vi "Launchtest.vi"(8 "error in (no error)":errorcluster, 11 "Operator name":string) -> (0 "error in (out)":errorcluster)   [LabVIEW 2024, in "LaunchTest.lvlib"]
doc: "This template is for the Queued Message Handler design pattern.\n\nThe Event Handling Loop generates messages based on user interface actions.\n\nThe Message Handling Loop processes messages generated by the Event Handling Loop, or by other messages. The messages are string values, so new messages can be added easily to the Message Cases case structure in the Message Handling Loop. Each message cluster can also provide an optional value for Message Data, which is a variant that can be converted to whatever message-specific data is required."
uses:
  LaunchTest.lvlib
  controls/Launch_UI Data.ctl
  PrivateControls/Launch_FGV_Queue_Control.ctl
  Test_2/TestMain2.vi
  <vilib>/Utility/error.llb/Error Cluster From Error Code.vi
  Launcher/MainLauncher.vi
  <vilib>/ErrorRing/Error Ring.xnode
  support/Message Queue/Launch_Message Queue.lvlib
  support/User Event - Stop/Launch_User Event - Stop.lvlib
  Launcher/Launcher_DTU.lvlib
  Test_2/Test_2.lvlib
  ADAM_DI/ADAM_DI.lvlib
panel:
  out "queue name 2":string
  out "queue name":string
  out "Display":string
  in  "Do Something Else <Replace Me>":bool
  in  "Do Something <Replace Me>":bool
  in  "Exit":bool
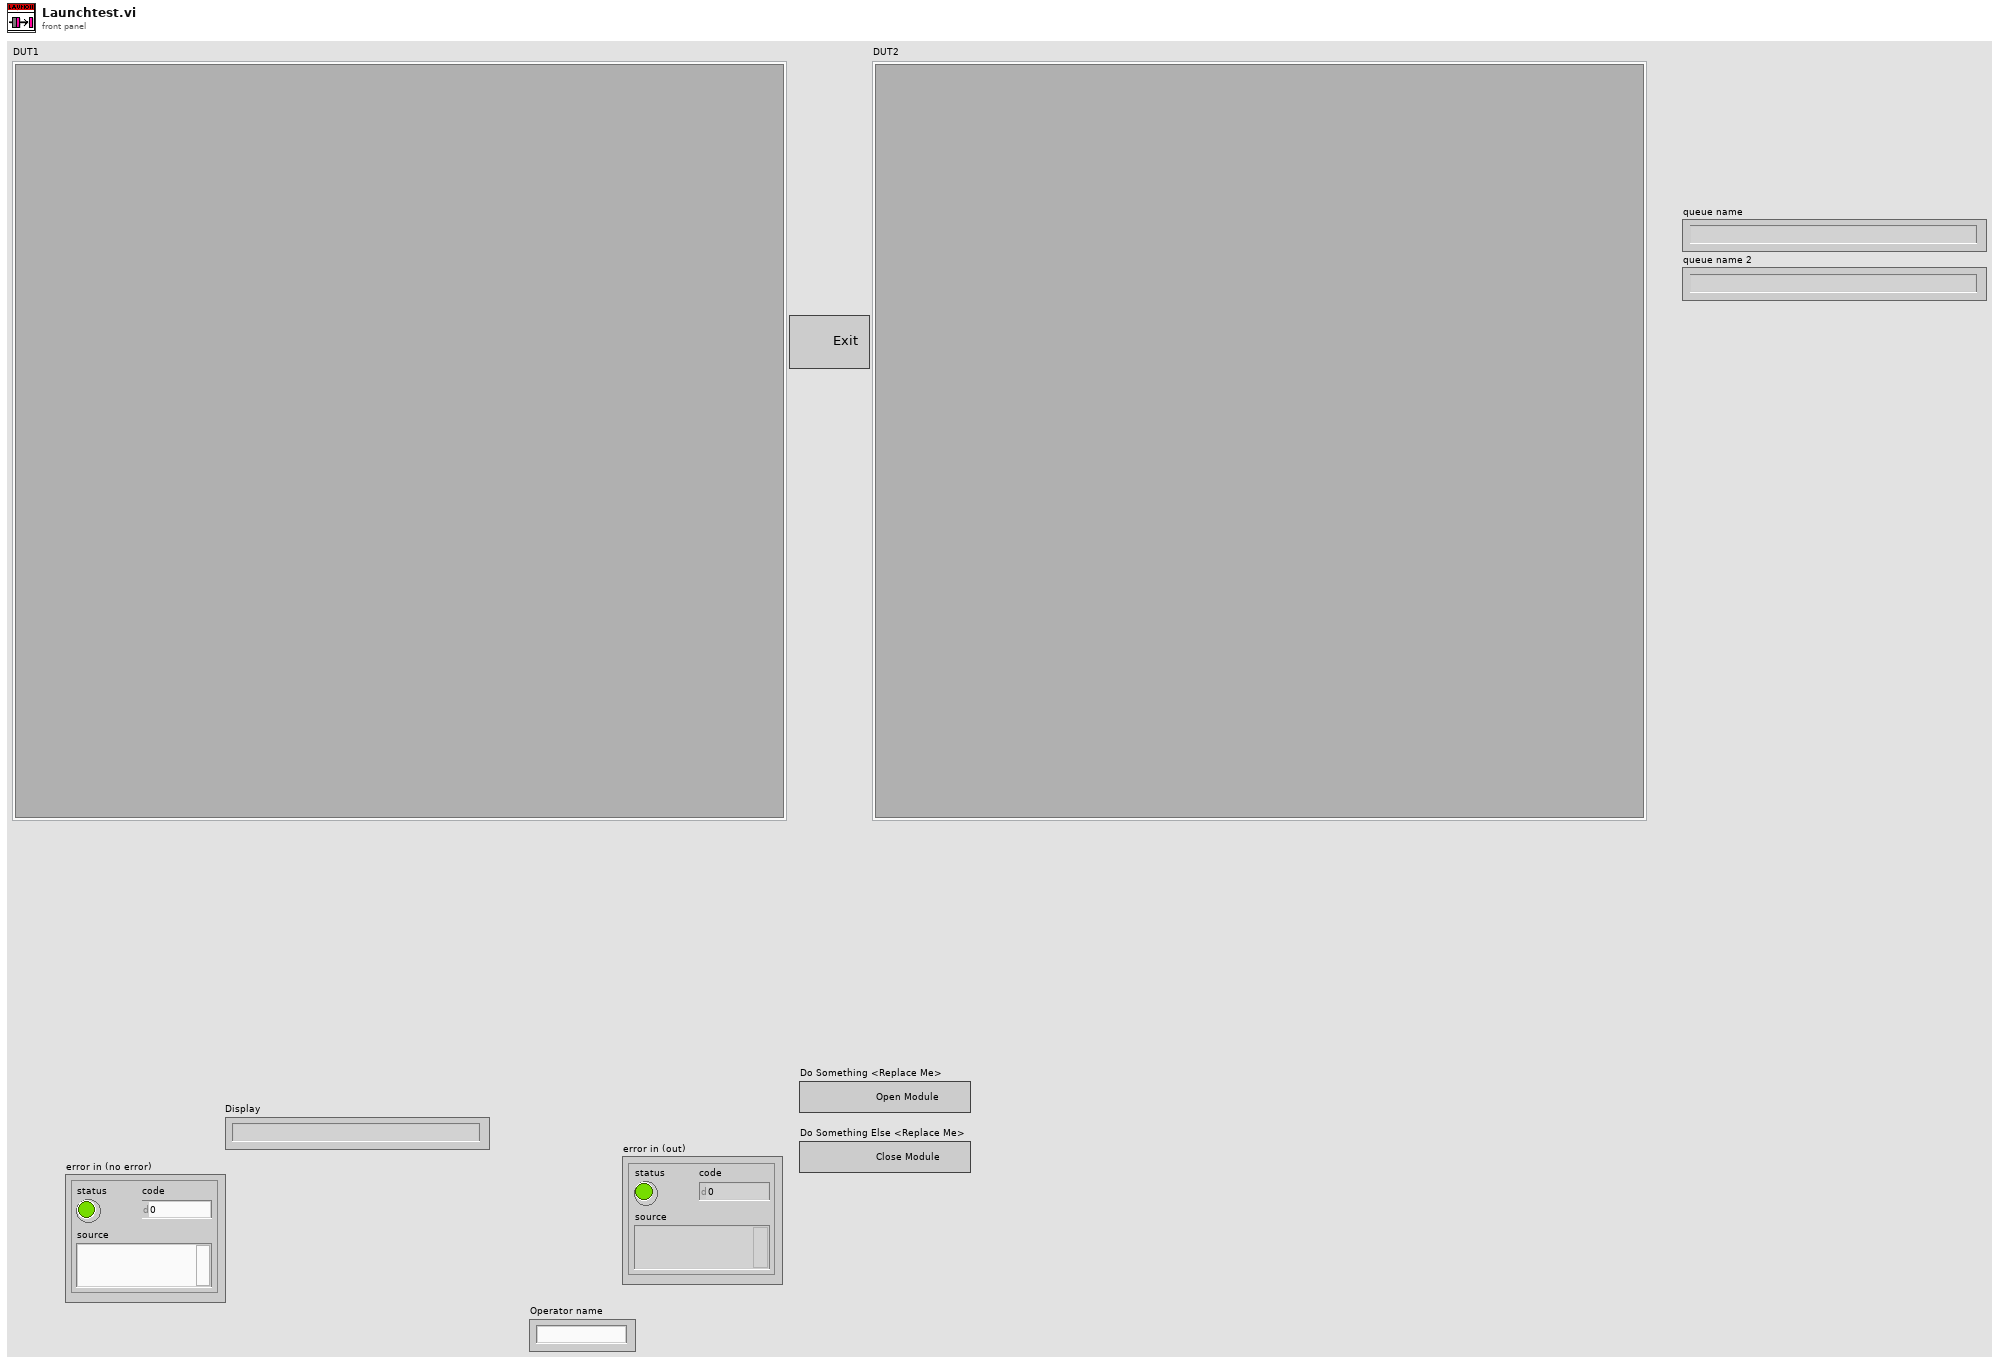
[diagram p1: front panel]
types:
  T1 = enum32{"Invalid", "Standard", "Closed", "Hidden", "Minimized", "Maximized"}
  T2 = typedef "LaunchTest.lvlib/Launch_FGV_Queue_Control.ctl" = enum16{"Release", "Get", "Set", "Flush"}
  T3 = typedef "LaunchTest.lvlib/Launch_UI Data.ctl" = cluster{"Launched?":bool, "Config":string, "Numeric <Replace Me>":dbl, "Operator":string, "Module path":path, "Config path":path, "Equip list":string[], "Test2_Q":refnum<queue>[], "CAMQ":refnum<queue>}
  T4 = typedef "LaunchTest.lvlib/Launch_Message Queue.lvlib/Launch_All Message Queues.ctl" = cluster{"UI":refnum<queue>, "QSM":refnum<queue>}
  T5 = enum16{"Read", "Write", "All_sections", "All_values", "Remove key&section"}
  T6 = cluster{"Message":string, "Message Data":variant}
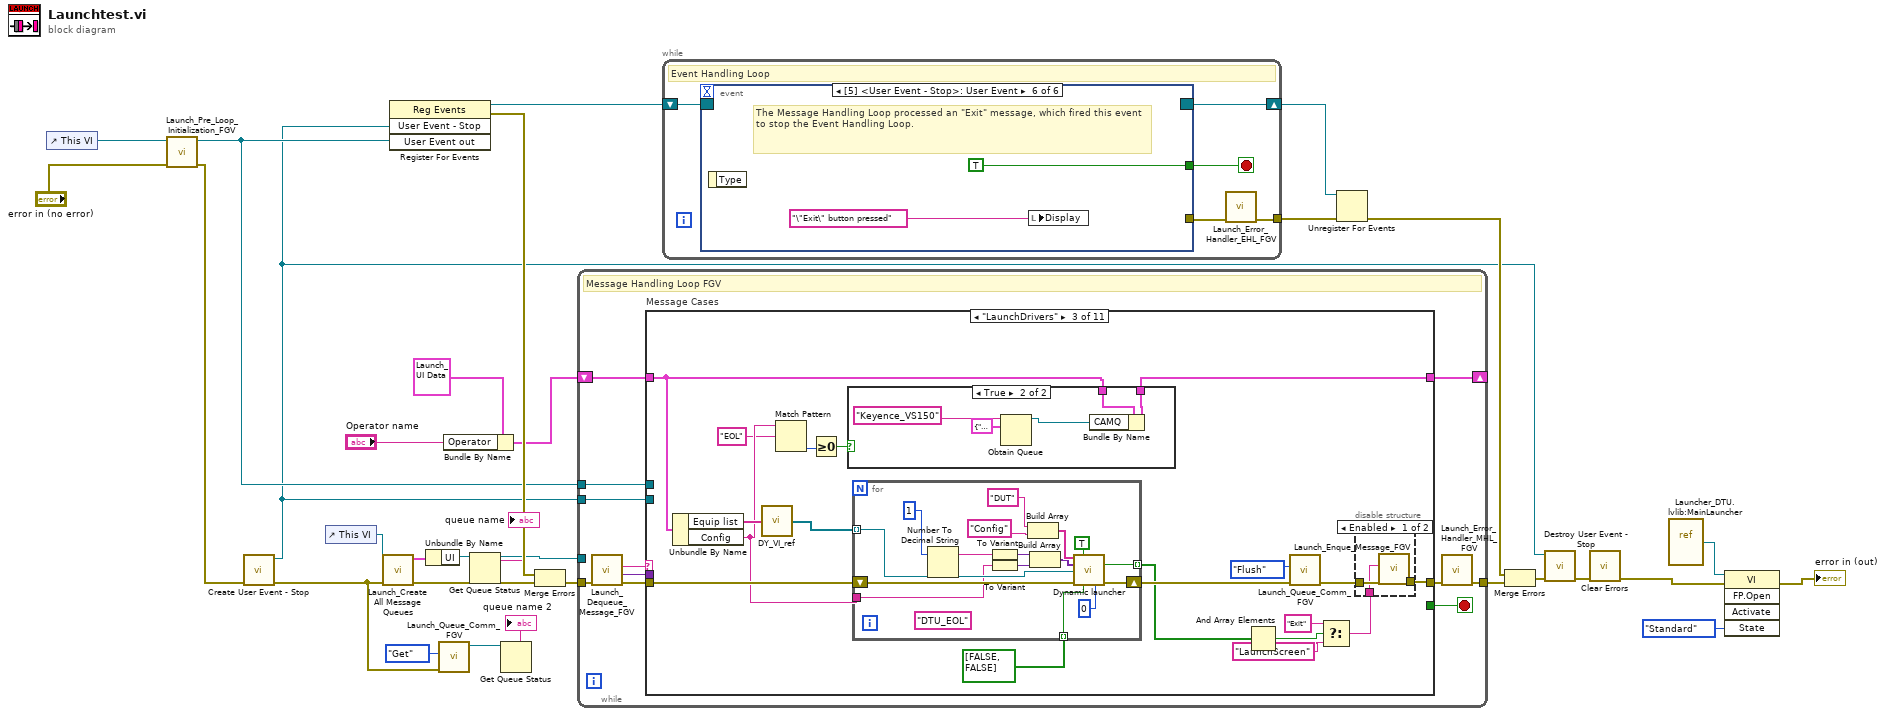
[diagram p0: block diagram]
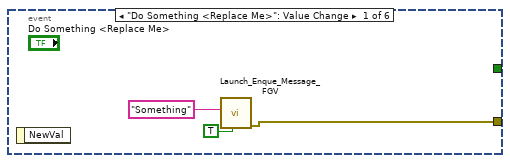
[diagram p2: hidden frame]
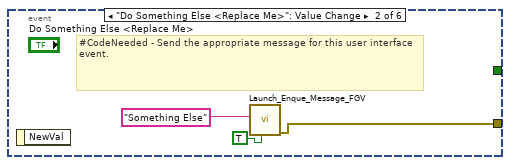
[diagram p3: hidden frame]
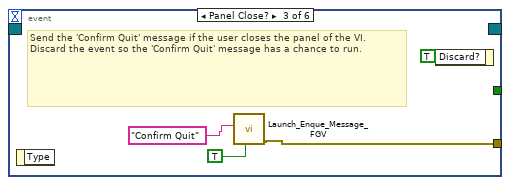
[diagram p4: hidden frame]
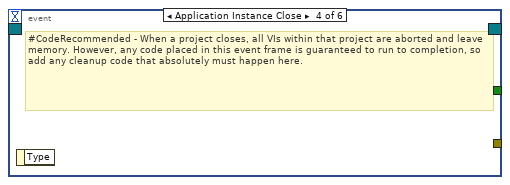
[diagram p5: hidden frame]
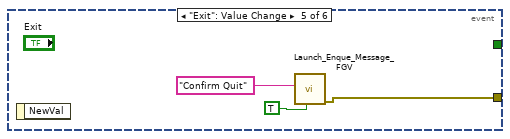
[diagram p6: hidden frame]
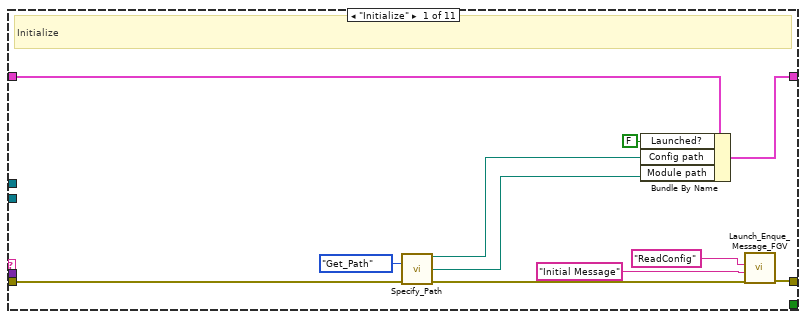
[diagram p7: hidden frame]
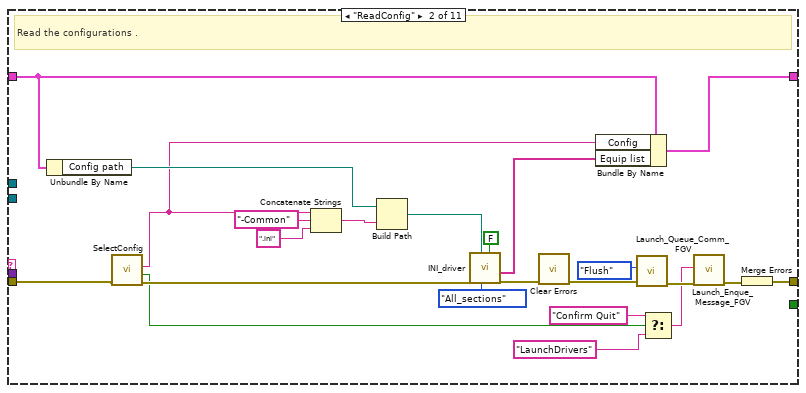
[diagram p8: hidden frame]
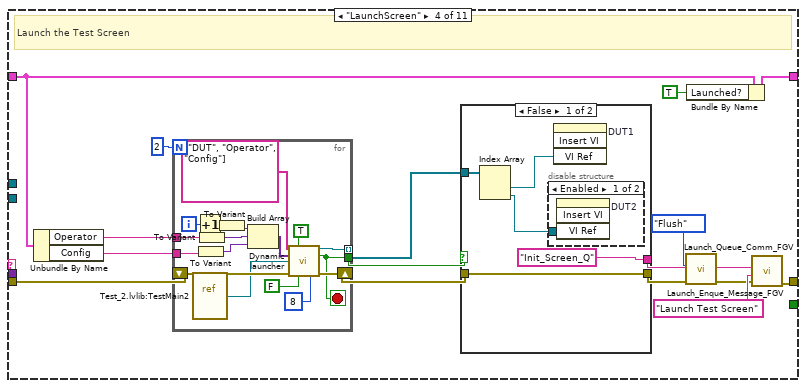
[diagram p11: hidden frame]
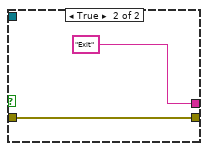
[diagram p13: hidden frame]
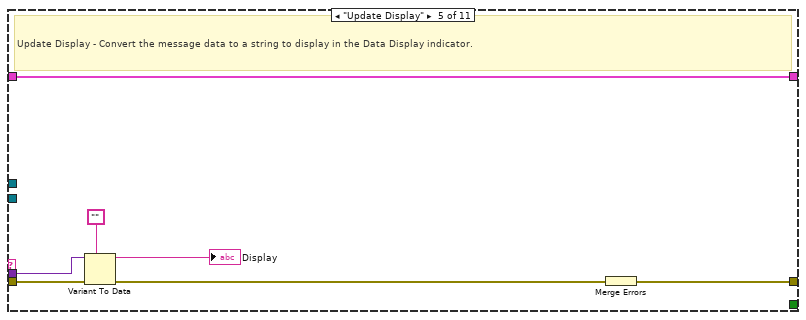
[diagram p14: hidden frame]
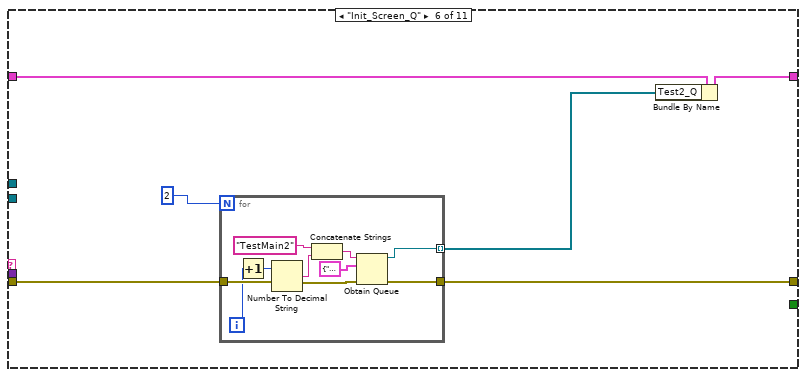
[diagram p15: hidden frame]
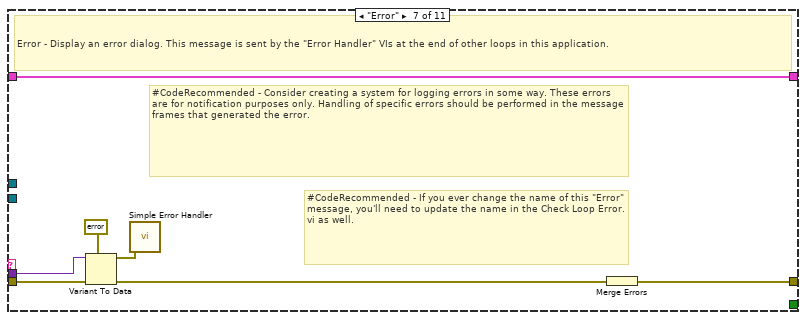
[diagram p16: hidden frame]
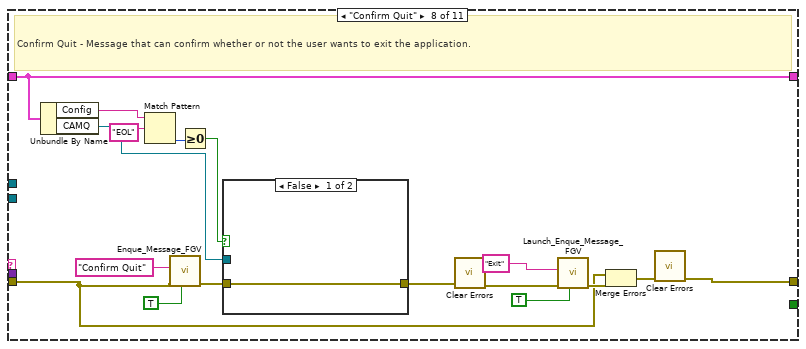
[diagram p17: hidden frame]
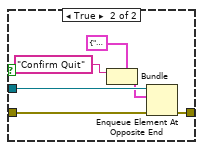
[diagram p18: hidden frame]
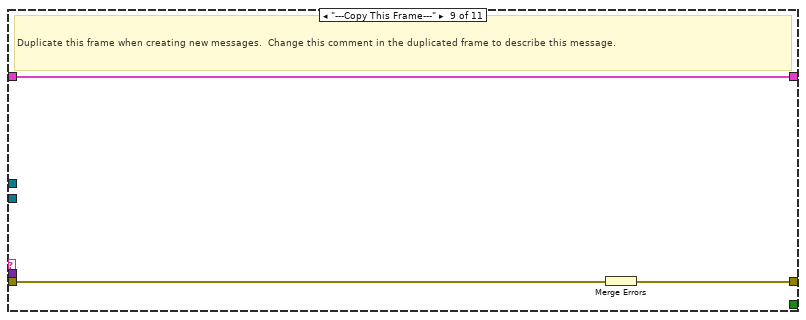
[diagram p19: hidden frame]
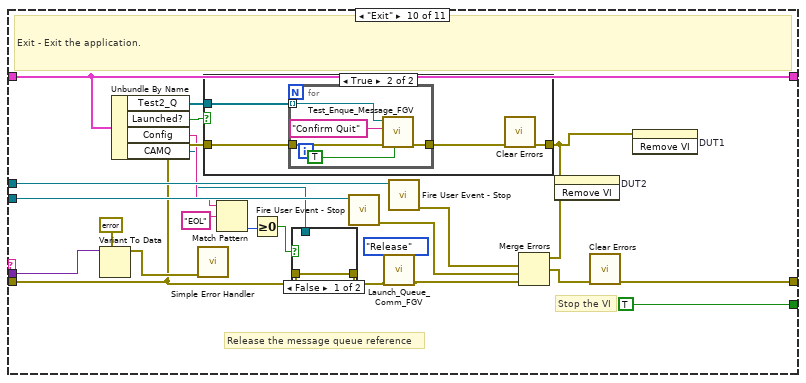
[diagram p20: hidden frame]
diagram:
  n1 = control-ref of="This VI"() -> (w19:refnum<vi>)
  n2 = call "Launch_Pre_Loop_Initialization_FGV.vi"("error in (no error)"="error in (no error)", "VI in"=w19) -> ("error out"=w17:errorcluster, "User Event out"=w8:refnum<user-event>)  [unwired: 8 in]
  n3 = call "Create User Event - Stop.vi"("error in (no error)"=w17) -> ("error out"=w12:errorcluster, "User Event - Stop"=w7:refnum<user-event>)  [unwired: 9 in]
  n4 = control-ref of="This VI"() -> (w15:refnum<vi>)
  n5 = call "Launch_Create All Message Queues.vi"("error in (no error)"=w12, "This VI"=w15) -> ("error out"=w31:errorcluster, "Message Queues out"=w30:T4)  [unwired: 8 in]
  n6 = register-events(w7, w8) -> (reference out=w22:refnum<event-registration>, error out=w20:errorcluster)  [unwired: 2 in]
  n7 = Unbundle By Name(w30) -> ("UI"=w28:refnum<queue>)
  n8 = call "Launch_Queue_Comm_FGV.vi"("error in (no error)"=w12, "Enum"=Launch_FGV_Queue_Control."Get") -> ("queue Out"=w10:refnum<queue>)  [unwired: 8 in, 1 out]
  n9 = Bundle By Name(cluster=T3 {"Launched?"=FALSE, "Config"="", "Numeric <Replace Me>"=0.0, "Operator"="", "Module path"=path "", "Config path"=path "", "Equip list"=[], "Test2_Q"=[], "CAMQ"=refnum} ("Data Cluster"), "Operator"="Operator name") -> (w2:T3)
  n10 = Get Queue Status(queue=w28) -> (queue out=w14:refnum<queue>, queue name=→"queue name":string)  [unwired: 2 in, 6 out]
  n11 = Get Queue Status(queue=w10) -> (queue name=→"queue name 2":string)  [unwired: 2 in, 7 out]
  n12 = Merge Errors(w20, w31) -> (w21:errorcluster)
  n13 = while {
    tunnel: w14 -> [_]
    shift-right: [w41] -> _
    shift-left: w2 -> [w42]
    tunnel: w8 -> [w39]
    tunnel: w21 -> [w38]
    tunnel: [w33] -> w29
    tunnel: w7 -> [w32]
    stop <- w40 stop-if-true
    # "Message Handling Loop FGV"
    n14 = call "Launch_Dequeue_Message_FGV.vi"("error in (no error)"=w38) -> ("error out"=w37:errorcluster, "Message Data"=w36:variant, "Message"=w35:string)  [unwired: 8 in]
    n15 = case "Message Cases" shown="\"LaunchDrivers\"" w35 {
      selector: w35 -> [_ _ _ _ _ _ _ _ _ _ w256]
      tunnel: w37 -> [w47 w61 w92 w137 w167 w175 w191 w201 w218 w230 _]
      tunnel: [w51 w76 w91 w135 w168 w173 w185 w203 w216 w227 w257] -> w34
      tunnel: w42 -> [w53 w70 w79 w136 w169 w174 w190 w196 w217 w228 w258]
      tunnel: [w52 w63 w78 w126 w169 w171 w190 w196 w217 w228 w258] -> w41
      tunnel: [_ _ _ _ _ _ _ _ _ TRUE _] -> w40
      tunnel: w36 -> [_ _ _ _ w166 _ w189 _ _ w236 _]
      tunnel: w39 -> [_ _ _ _ _ _ _ _ _ w239 _]
      tunnel: w32 -> [_ _ _ _ _ _ _ _ _ w233 _]
      frame "Initialize" {
        # "Initialize"
        n16 = call "Specify_Path.vi"("Path_Enum"=enum16{"Find_Path", "Get_Path"}."Get_Path", "error in (no error)"=w47) -> ("Configurations"=w44:path, "Modules path"=w43:path, "error out"=w46:errorcluster)  [unwired: 6 in, 5 out]
        n17 = Bundle By Name(cluster=w53, "Launched?"=FALSE, "Config path"=w44, "Module path"=w43) -> (w52:T3)
        n18 = call "Launch_Enque_Message_FGV.vi"("error in (no error)"=w46, "Message Data"="Initial Message" ("Initial Message"), "Message"="ReadConfig") -> ("error out"=w51:errorcluster)  [unwired: 8 in]
      }
      frame "ReadConfig" {
        # "Read the configurations ."
        n19 = Unbundle By Name(w70) -> ("Config path"=w68:path)
        n20 = call "SelectConfig.vi"("error in"=w61) -> ("error constant"=w60:errorcluster, "Cancel"=w59:bool, "Config"=w54:string)  [unwired: 8 in]
        n21 = Concatenate Strings(w54, "-Common", ".ini" ("string")) -> (w69:string)
        n22 = Build Path(base path=w68, name or relative path=w69) -> (appended path=w66:path)
        n23 = call "INI_driver.vi"("create file if necessary (T)"=FALSE, "Enum"=T5."All_sections", "instrument file path"=w66, "error in (no error)"=w60) -> ("error out"=w67:errorcluster, "section names"=w62:string[])  [unwired: 4 in, 2 out]
        n24 = call <vilib>:"Clear Errors.vi"("error in (no error)"=w67) -> ("error out"=w55:errorcluster)  [unwired: 5 in, 1 out]
        n25 = Bundle By Name(cluster=w70, "Config"=w54, "Equip list"=w62) -> (w63:T3)
        n26 = call "Launch_Queue_Comm_FGV.vi"("error in (no error)"=w55, "Enum"=Launch_FGV_Queue_Control."Flush") -> ("error Out"=w74:errorcluster)  [unwired: 8 in, 1 out]
        n27 = Select(t="Confirm Quit", s=w59, f="LaunchDrivers") -> (s? t:f=w57:string)
        n28 = call "Launch_Enque_Message_FGV.vi"("error in (no error)"=w74, "Message"=w57) -> ("error out"=w75:errorcluster)  [unwired: 9 in]
        n29 = Merge Errors(w75) -> (w76:errorcluster)
      }
      frame "LaunchDrivers" {
        n30 = Unbundle By Name(w79) -> ("Equip list"=w85:string[], "Config"=w83:string)
        n31 = call "DY_VI_ref.vi"("EQUIP LIST"=w85) -> ("VI_ref"=w84:refnum<vi>[])
        n32 = Match Pattern(string=w83, regular expression="EOL" ("search string")) -> (offset past match=w81:i32)  [unwired: 1 in, 3 out]
        n33 = Greater Or Equal To 0?(x=w81) -> (x >= 0?=w80:bool)
        n34 = case shown="True" w80 {
          tunnel: w79 -> [w96 w99]
          tunnel: [w96 w98] -> w78
          frame False {
          }
          frame True {
            n35 = Obtain Queue(name (unnamed)="Keyence_VS150", element data type=T6 {"Message"="", "Message Data"=variant} ("Message Cluster")) -> (queue out=w97:refnum<queue>)  [unwired: 3 in, 2 out]
            n36 = Bundle By Name(cluster=w99, "CAMQ"=w97) -> (w98:T3)
          }
        }
        n37 = for {
          shift-right: [w121] -> w90
          shift-left: w92 -> [w113]
          tunnel: [w120] -> w88 mode=indexing
          tunnel: w84 -> [w110] mode=indexing
          tunnel: w83 -> [w109]
          tunnel: bool[] [FALSE, FALSE] ("Open FP") -> [w106] mode=indexing
          (unwired) "DTU_EOL"
          n38 = Number To Decimal String(number=1) -> (decimal integer string=w108:string)  [unwired: 1 in]
          n39 = To Variant(anything=w108) -> (Variant=w115:variant)
          n40 = To Variant(anything=w109) -> (Variant=w114:variant)
          n41 = Build Array("DUT", "Config") -> (w117:string[])
          n42 = Build Array(w115, w114) -> (w116:variant[])
          n43 = call "Dynamic launcher.vi"("element"=w117, "Clone ?"=TRUE, "Value"=w116, "VI Refnum"=w110, "error in (no error)"=w113, "Open FP"=w106, "options"=0) -> ("Failed"=w120:bool, "error out"=w121:errorcluster)  [unwired: 6 in, 1 out]
        }
        n44 = And Array Elements(Boolean array=w88) -> (logical AND=w87:bool)
        n45 = call "Launch_Queue_Comm_FGV.vi"("error in (no error)"=w90, "Enum"=Launch_FGV_Queue_Control."Flush") -> ("error Out"=w95:errorcluster)  [unwired: 8 in, 1 out]
        n46 = Select(t="Exit" ("f"), s=w87, f="LaunchScreen") -> (s? t:f=w89:string)
        n47 = disable-structure shown="Enabled" {
          disable-tunnel: w95 -> [w104 w105]
          disable-tunnel: [w103 w105] -> w91
          disable-tunnel: w89 -> [w102 _]
          frame Enabled {
            n48 = call "Launch_Enque_Message_FGV.vi"("error in (no error)"=w104, "Message"=w102) -> ("error out"=w103:errorcluster)  [unwired: 9 in]
          }
          frame Disabled {
          }
        }
      }
      frame "LaunchScreen" {
        # "Launch the Test Screen"
        n49 = Unbundle By Name(w136) -> ("Operator"=w124:string, "Config"=w122:string)
        n50 = for {
          N: 2 -> [_]
          shift-right: [w161] -> w134
          shift-left: w137 -> [w162]
          tunnel: [w155] -> w131
          tunnel: [w154] -> w129 mode=indexing
          tunnel: w124 -> [w148]
          tunnel: w122 -> [w147]
          i -> [w160]
          stop <- w155 stop-if-true
          n51 = vi-ref "Test_2.lvlib:TestMain2.vi"() -> (w149:refnum<vi>)
          n52 = Increment(x=w160) -> (x+1=w159:i32)
          n53 = To Variant(anything=w147) -> (Variant=w146:variant)
          n54 = To Variant(anything=w148) -> (Variant=w150:variant)
          n55 = To Variant(anything=w159) -> (Variant=w158:variant)
          n56 = Build Array(w158, w150, w146) -> (w157:variant[])
          n57 = call "Dynamic launcher.vi"("element"=string[] ["DUT", "Operator", "Config"], "Clone ?"=TRUE, "Value"=w157, "VI Refnum"=w149, "error in (no error)"=w162, "Open FP"=FALSE, "options"=8) -> ("reference out"=w154:refnum<vi>, "Failed"=w155:bool, "error out"=w161:errorcluster)  [unwired: 6 in]
        }
        n58 = case shown="False" w131 {
          tunnel: w134 -> [w142 w145]
          tunnel: [w142 w145] -> w133
          tunnel: ["Init_Screen_Q" ("Message") "Exit" ("Message")] -> w130
          tunnel: w129 -> [w140 _]
          frame False {
            n59 = Index Array(array=w140) -> (element #1=w139:refnum<vi>, element #2=w138:refnum<vi>)  [unwired: 2 in]
            n60 = disable-structure shown="Enabled" {
              disable-tunnel: w138 -> [w143 _]
              frame Enabled {
                n61 = invoke on="DUT2" class="SubPnl" method="Insert VI"("VI Ref"=w143) -> ()  [unwired: 3 in, 4 out]
              }
              frame Disabled {
              }
            }
            n62 = invoke on="DUT1" class="SubPnl" method="Insert VI"("VI Ref"=w139) -> ()  [unwired: 3 in, 4 out]
          }
          frame True {
          }
        }
        n63 = call "Launch_Queue_Comm_FGV.vi"("error in (no error)"=w133, "Enum"=Launch_FGV_Queue_Control."Flush") -> ("error Out"=w128:errorcluster)  [unwired: 8 in, 1 out]
        n64 = Bundle By Name(cluster=w136, "Launched?"=TRUE) -> (w126:T3)
        n65 = call "Launch_Enque_Message_FGV.vi"("error in (no error)"=w128, "Message Data"="Launch Test Screen" ("Message"), "Message"=w130) -> ("error out"=w135:errorcluster)  [unwired: 8 in]
      }
      frame "Update Display" {
        # "Update Display - Convert the message data to a string to display in the Data Display indicator."
        n66 = Variant To Data(error in=w167, type="", Variant=w166) -> (data=→"Display":string, error out=w164:errorcluster)
        n67 = Merge Errors(w164) -> (w168:errorcluster)
      }
      frame "Init_Screen_Q" {
        n68 = for {
          N: 2 -> [_]
          tunnel: w175 -> [w184]
          tunnel: [w183] -> w173
          tunnel: [w177] -> w170 mode=indexing
          i -> [w179]
          n69 = Increment(x=w179) -> (x+1=w176:i32)
          n70 = Number To Decimal String(number=w176) -> (decimal integer string=w178:string)  [unwired: 1 in]
          n71 = Concatenate Strings("TestMain2", w178) -> (w181:string)
          n72 = Obtain Queue(name (unnamed)=w181, element data type=T6 {"Message"="", "Message Data"=variant} ("notification"), error in (no error)=w184) -> (queue out=w177:refnum<queue>, error out=w183:errorcluster)  [unwired: 2 in, 1 out]
        }
        n73 = Bundle By Name(cluster=w174, "Test2_Q"=w170) -> (w171:T3)
      }
      frame "Error" {
        # "#CodeRecommended - If you ever change the name of this \"Error\" message, you'll need to update the name in the Check Loop Error.vi as well."
        # "#CodeRecommended - Consider creating a system for logging errors in some way. These errors are for notification purposes only. Handling of specific errors should be performed in the message frames that generated the error."
        # "Error - Display an error dialog. This message is sent by the \"Error Handler\" VIs at the end of other loops in this application."
        n74 = Variant To Data(error in=w191, type=errorcluster {"status"=FALSE, "code"=0, "source"=""} ("error constant"), Variant=w189) -> (data=w187:errorcluster, error out=w186:errorcluster)
        n75 = call <vilib>:"Simple Error Handler.vi"("error in (no error)"=w187) -> ()  [unwired: 4 in, 5 out]
        n76 = Merge Errors(w186) -> (w185:errorcluster)
      }
      frame "Confirm Quit" {
        # "Confirm Quit - Message that can confirm whether or not the user wants to exit the application."
        n77 = Unbundle By Name(w196) -> ("Config"=w195:string, "CAMQ"=w193:refnum<queue>)
        n78 = Match Pattern(string=w195, regular expression="EOL" ("search string")) -> (offset past match=w197:i32)  [unwired: 1 in, 3 out]
        n79 = call "Enque_Message_FGV.vi"("Priority"=TRUE ("Priority Message? (F)"), "error in (no error)"=w201, "Message"="Confirm Quit") -> ("error out"=w200:errorcluster)  [unwired: 8 in]
        n80 = Greater Or Equal To 0?(x=w197) -> (x >= 0?=w192:bool)
        n81 = case shown="False" w192 {
          tunnel: w200 -> [w209 w215]
          tunnel: [w209 w214] -> w194
          tunnel: w193 -> [_ w213]
          frame False {
          }
          frame True {
            n82 = Bundle(cluster=T6 {"Message"="", "Message Data"=variant} ("element"), "Message"="Confirm Quit") -> (w211:T6)  [unwired: 1 in]
            n83 = Enqueue Element At Opposite End(queue=w213, element=w211, error in (no error)=w215) -> (error out=w214:errorcluster)  [unwired: 1 in, 2 out]
          }
        }
        n84 = call <vilib>:"Clear Errors.vi"("error in (no error)"=w194) -> ("error out"=w204:errorcluster)  [unwired: 5 in, 1 out]
        n85 = call "Launch_Enque_Message_FGV.vi"("Priority"=TRUE ("Priority Message? (F)"), "error in (no error)"=w204, "Message"="Exit") -> ("error out"=w207:errorcluster)  [unwired: 8 in]
        n86 = Merge Errors(w201, w207) -> (w208:errorcluster)
        n87 = call <vilib>:"Clear Errors.vi"("error in (no error)"=w208) -> ("error out"=w203:errorcluster)  [unwired: 5 in, 1 out]
      }
      frame "---Copy This Frame---" {
        # "Duplicate this frame when creating new messages.  Change this comment in the duplicated frame to describe this message."
        n88 = Merge Errors(w218) -> (w216:errorcluster)
      }
      frame "Exit" {
        # "Stop the VI"
        # "Release the message queue reference"
        # "Exit - Exit the application."
        n89 = Variant To Data(type=errorcluster {"status"=FALSE, "code"=0, "source"=""} ("error constant"), Variant=w236) -> (data=w237:errorcluster)  [unwired: 1 in, 1 out]
        n90 = Unbundle By Name(w228) -> ("Test2_Q"=w225:refnum<queue>[], "Launched?"=w229:bool, "Config"=w222:string, "CAMQ"=w220:refnum<queue>)
        n91 = call <vilib>:"Simple Error Handler.vi"("error in (no error)"=w237) -> ()  [unwired: 4 in, 5 out]
        n92 = case shown="True" w229 {
          tunnel: w230 -> [w246 w250]
          tunnel: [w246 w247] -> w226
          tunnel: w225 -> [_ w249]
          frame False {
          }
          frame True {
            n93 = for {
              tunnel: w250 -> [w255]
              tunnel: [w254] -> w248
              tunnel: w249 -> [w252] mode=indexing
              n94 = call "Test_Enque_Message_FGV.vi"("Priority"=TRUE, "error in (no error)"=w255, "Message"="Confirm Quit", "queue in"=w252) -> ("error out"=w254:errorcluster)  [unwired: 7 in]
            }
            n95 = call <vilib>:"Clear Errors.vi"("error in (no error)"=w248) -> ("error out"=w247:errorcluster)  [unwired: 5 in, 1 out]
          }
        }
        n96 = Match Pattern(string=w222, regular expression="EOL" ("search string")) -> (offset past match=w223:i32)  [unwired: 1 in, 3 out]
        n97 = Greater Or Equal To 0?(x=w223) -> (x >= 0?=w219:bool)
        n98 = case shown="False" w219 {
          tunnel: w230 -> [w242 w245]
          tunnel: [w242 w244] -> w221
          tunnel: w220 -> [_ w243]
          frame False {
          }
          frame True {
            n99 = Release Queue(queue=w243, error in (no error)=w245) -> (error out=w244:errorcluster)  [unwired: 1 in, 2 out]
          }
        }
        n100 = call "Fire User Event - Stop.vi"("User Event - Stop"=w233) -> ("error out"=w231:errorcluster)  [unwired: 10 in]
        n101 = call "Launch_Queue_Comm_FGV.vi"("error in (no error)"=w221, "Enum"=Launch_FGV_Queue_Control."Release") -> ("error Out"=w234:errorcluster)  [unwired: 8 in, 1 out]
        n102 = call "Fire User Event - Stop.vi"("User Event - Stop"=w239) -> ("error out"=w232:errorcluster)  [unwired: 10 in]
        n103 = Merge Errors(w226, w232, w231, w234) -> (w240:errorcluster)
        n104 = invoke on="DUT2" class="SubPnl" method="Remove VI"(error in=w226) -> ()  [unwired: 2 in, 3 out]
        n105 = call <vilib>:"Clear Errors.vi"("error in (no error)"=w240) -> ("error out"=w227:errorcluster)  [unwired: 5 in, 1 out]
        n106 = invoke on="DUT1" class="SubPnl" method="Remove VI"(error in=w226) -> ()  [unwired: 2 in, 3 out]
      }
      frame Default {
        # "'Default' case only runs if there is a message that isn't defined in any of the other cases.  Output a programming error."
        n107 = xnode "Error Ring"("parameter 0"=w256) -> ("error out"=w257:errorcluster)
      }
    }
    n108 = call "Launch_Error_Handler_MHL_FGV.vi"("error in (no error)"=w34) -> ("error Out"=w33:errorcluster)  [unwired: 10 in]
  }
  n109 = while {
    shift-right: [w269] -> w25
    shift-left: w22 -> [w270]
    tunnel: [w266] -> w23
    stop <- w268 stop-if-true
    # "Event Handling Loop"
    n110 = event shown="[5] <User Event - Stop>: User Event" {
      selector: w270 -> [_ _ _ _ _ _]
      dyn-events: [_ _ _ _ _ _] -> w269
      timeout: _ -> [_ _ _ _ _ _]
      tunnel: [_ _ _ _ _ TRUE ("Discard?")] -> w268
      tunnel: [w272 w274 w279 _ w283 _] -> w267
      event "Do Something <Replace Me>": Value Change {
        n111 = event-data() -> ()  [unwired: 1 in, 1 out]
        n112 = call "Launch_Enque_Message_FGV.vi"("Priority"=TRUE ("Priority Message? (F)"), "Message"="Something") -> ("error out"=w272:errorcluster)  [unwired: 9 in]
      }
      event "Do Something Else <Replace Me>": Value Change {
        # "#CodeNeeded - Send the appropriate message for this user interface event."
        n113 = event-data() -> ()  [unwired: 1 in, 1 out]
        n114 = call "Launch_Enque_Message_FGV.vi"("Priority"=TRUE ("Priority Message? (F)"), "Message"="Something Else") -> ("error out"=w274:errorcluster)  [unwired: 9 in]
      }
      event Panel Close? {
        # "Send the 'Confirm Quit' message if the user closes the panel of the VI. Discard the event so the 'Confirm Quit' message has a chance to run."
        n115 = event-data() -> ()  [unwired: 1 in, 1 out]
        n116 = call "Launch_Enque_Message_FGV.vi"("Priority"=TRUE ("Priority Message? (F)"), "Message"="Confirm Quit") -> ("error out"=w279:errorcluster)  [unwired: 9 in]
        n117 = event-data("Discard?"=TRUE) -> ()  [unwired: 1 in, 1 out]
      }
      event Application Instance Close {
        # "#CodeRecommended - When a project closes, all VIs within that project are aborted and leave memory. However, any code placed in this event frame is guaranteed to run to completion, so add any cleanup code that absolutely must happen here."
        n118 = event-data() -> ()  [unwired: 1 in, 1 out]
      }
      event "Exit": Value Change {
        n119 = event-data() -> ()  [unwired: 1 in, 1 out]
        n120 = call "Launch_Enque_Message_FGV.vi"("Priority"=TRUE ("Priority Message? (F)"), "Message"="Confirm Quit") -> ("error out"=w283:errorcluster)  [unwired: 9 in]
      }
      event User Event {
        # "The Message Handling Loop processed an \"Exit\" message, which fired this event to stop the Event Handling Loop."
        n121 = event-data() -> ()  [unwired: 1 in, 1 out]
        n122 = local write "Display"("\"Exit\" button pressed" ("VI Stopped")) -> ()
      }
    }
    n123 = call "Launch_Error_Handler_EHL_FGV.vi"("error in (no error)"=w267) -> ("error Out"=w266:errorcluster)  [unwired: 10 in]
  }
  n124 = Unregister For Events(event registration refnum=w25, error in=w23) -> (error out=w26:errorcluster)
  n125 = Merge Errors(w26, w29) -> (w27:errorcluster)
  n126 = call "Destroy User Event - Stop.vi"("error in (no error)"=w27, "User Event - Stop"=w7) -> ("error out"=w16:errorcluster)  [unwired: 9 in]
  n127 = call <vilib>:"Clear Errors.vi"("error in (no error)"=w16) -> ("error out"=w6:errorcluster)  [unwired: 5 in, 1 out]
  n128 = vi-ref "Launcher_DTU.lvlib:MainLauncher.vi"() -> (w4:refnum<vi>)
  n129 = invoke class="VI" method="FP.Open"(reference=w4, error in=w6, "State"=T1."Standard") -> (error out=→"error in (out)":errorcluster)  [unwired: 2 in, 4 out]
